vi "Write VI Refnum Actor Core.vi"(8 "error in (no error)":errorcluster, 10 "VI Refnum Actor Core":refnum<vi>, 11 "Coins in":refnum<class "Coins.lvclass">) -> (0 "error out":errorcluster, 3 "Coins out":refnum<class "Coins.lvclass">)   [LabVIEW 2020, in "Coins.lvlib" / "Coins.lvclass"]
uses:
  Coins.lvclass
  Coins.lvclass/Coins.ctl
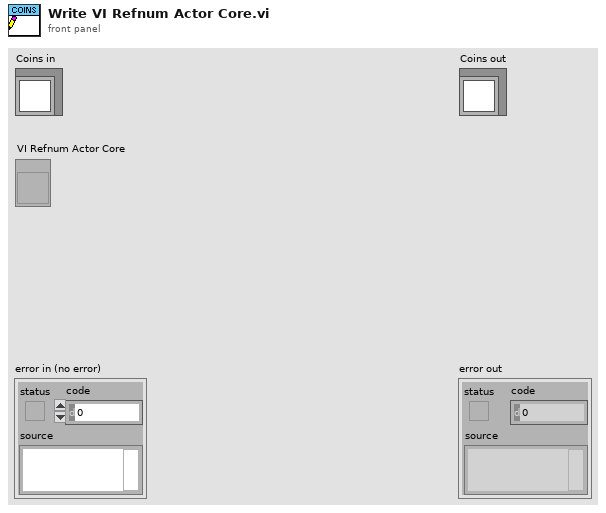
[diagram p1: front panel]
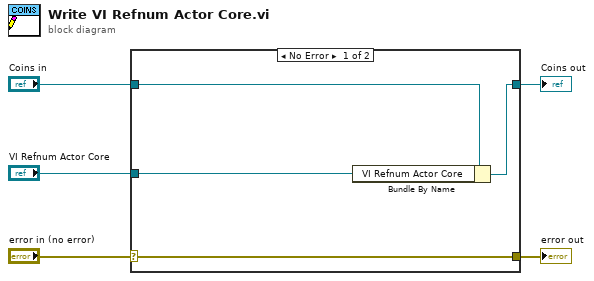
[diagram p0: block diagram]
diagram:
  n1 = case shown="No Error" "error in (no error)" {
    selector: "error in (no error)" -> [w9 w10]
    tunnel: [w9 w10] -> w4
    tunnel: [w7 w11] -> w2
    tunnel: "Coins in" -> [w8 w11]
    tunnel: "VI Refnum Actor Core" -> [w6 _]
    frame No Error {
      n2 = Bundle By Name(cluster=w8, "VI Refnum Actor Core"=w6) -> (w7:refnum<class "Coins.lvclass">)
    }
    frame Error {
    }
  }
  "error out" <- w4
  "Coins out" <- w2
